vi "FFT and Power Spectrum Units.vi"() -> ()   [LabVIEW 2020]
doc: "This is an interactive example which allows you to explore the subject of FFT and spectrum output units.\n\nThe input signal to the FFT-based VIs is constructed as a single frequency component with a DC offset so that both the DC and non-DC amplitudes can be easily verified."
uses:
  <vilib>/measure/maspectr.llb/Power Spectrum and PSD Export Mode.ctl
  <vilib>/Analysis/2dsp.llb/Real FFT.vi
  <vilib>/Analysis/2dsp.llb/Power Spectrum (DBL).vi
  <vilib>/measure/maspectr.llb/FFT Power Spectrum and PSD for 1 Chan.vi
  <vilib>/measure/maspectr.llb/FFT Spectrum (Mag-Phase) for 1 Chan.vi
  <vilib>/measure/maspectr.llb/FFT Spectrum (Real-Im) for 1 Chan.vi
  <vilib>/Analysis/NI_AALPro.lvlib
  <vilib>/gmath/NI_Gmath.lvlib
  <vilib>/measure/NI_MAPro.lvlib
  <vilib>/measure/NI_MABase.lvlib
panel:
  in  "Instructions":string="Overview: Shows the propagation of units through FFT-based measurements. \nRequirements: LabVIEW Full Development System\nInstructions:\n1. Run the VI.  Make sure sine frequency is \"on bin\" by making sure it is an integer multiple of df = sample rate/number of samples.\n2. In the spectrum units table, click in either the Unit (DC) column or the Unit (freq > 0) column of any function row to validate agreement between the text formula in the cell and the spectral plot component.\n3. Click Stop to stop the VI."
  out "axis dx":dbl=1.0
  in  "x axis unit":u16(ring) items=["bin index", "frequency in Hz"]
  out "phase[k] in deg":dbl=-89.99999999994303
  out "phase spectrum":dbl[](array[numeric])
  out "k = bin index = f/df":dbl=10.0
  out "df (Hz) = Fs/N":dbl=20.0
  in  "Stop":bool
  in  "V":dbl=2.0
  out "spectrum units table":string[][](table)=[["FFT", "N * V", "N/2 * Vpk"], ["Power Spectrum", "V^2", "1/2 * Vrms^2"], ["Auto Power Spectrum", "V^2", "Vrms^2"], ["Amplitude and Phase Spectrum", "V", "Vrms"], ["FFT Power Spectrum", "V^2", "Vrms^2"], ["FFT Power Spectral Density", "V^2/Hz", "Vrms^2/Hz"], ["FFT Spectrum (Mag-Phase)", "V", "Vrms"], ["FFT Spectrum (Real-Imag)", "V", "Vrms"]]
  out "Vrms":dbl=2.1213203435596424
  out "X[0 or k]":dbl=150.0
  out "spectral plot":cluster{"t":dbl, "t":dbl, "magnitude":dbl[]}(graph)={"t"=0.0, "t"=1.0, "magnitude"=[]}
  out "time domain signal":waveform(dbl)(graph)={"t0"=timestamp(14.25 s since 1904-01-01), "dt"=0.0005, "Y"=[]}
  in  "Fs, sample rate":dbl=2000.0
  in  "N":dbl=100.0
  in  "sine frequency":dbl=200.0
  in  "Vpk":dbl=3.0
  # "Selecting either of the Unit columns in the table will place a cursor on the corresponding component in the plot, and the Y value of that component is displayed in the X[0 or k] indicator below."
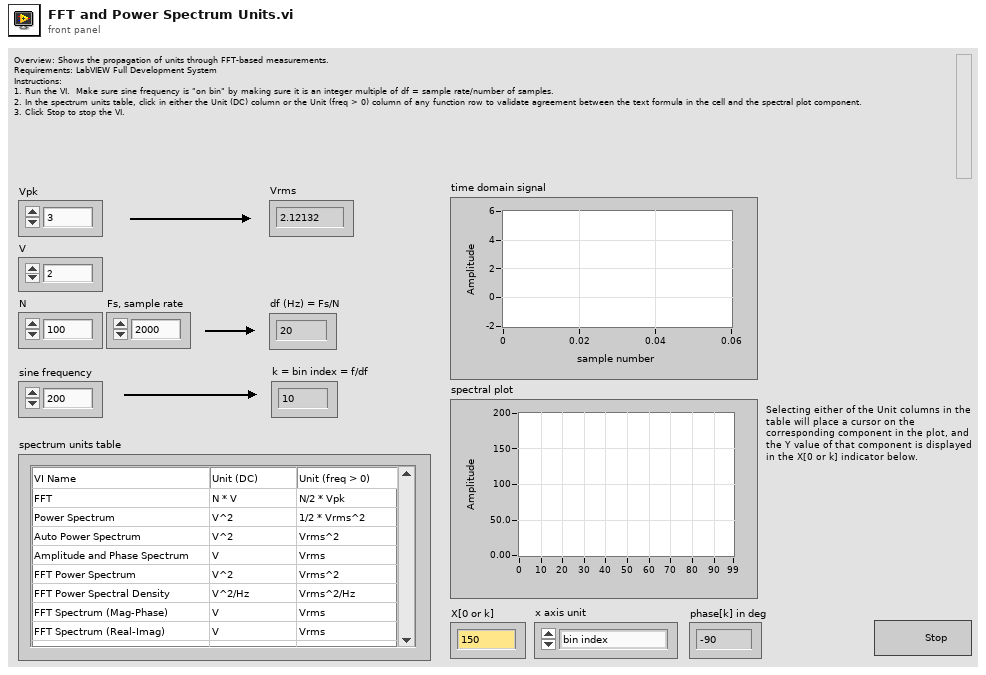
[diagram p1: front panel]
types:
  T1 = enum16{"None ", "Hanning", "Hamming", "Blackman-Harris", "Exact Blackman", "Blackman", "Flat Top", "4 Term B-Harris ", "7 Term B-Harris", "Low Sidelobe"}
  T2 = cluster{"dB On (F)":bool, "unwrap phase (F)":bool, "convert to degree (F)":bool}
  T3 = typedef "LVRowAndColumnTypeDef.ctl" = cluster{"Row":i32, "Column":i32}
  T4 = typedef "NI_MAPro.lvlib/Power Spectrum and PSD Export Mode.ctl" = u16
  T5 = cluster{"f0":dbl, "df":dbl, "imaginary part":dbl[]}
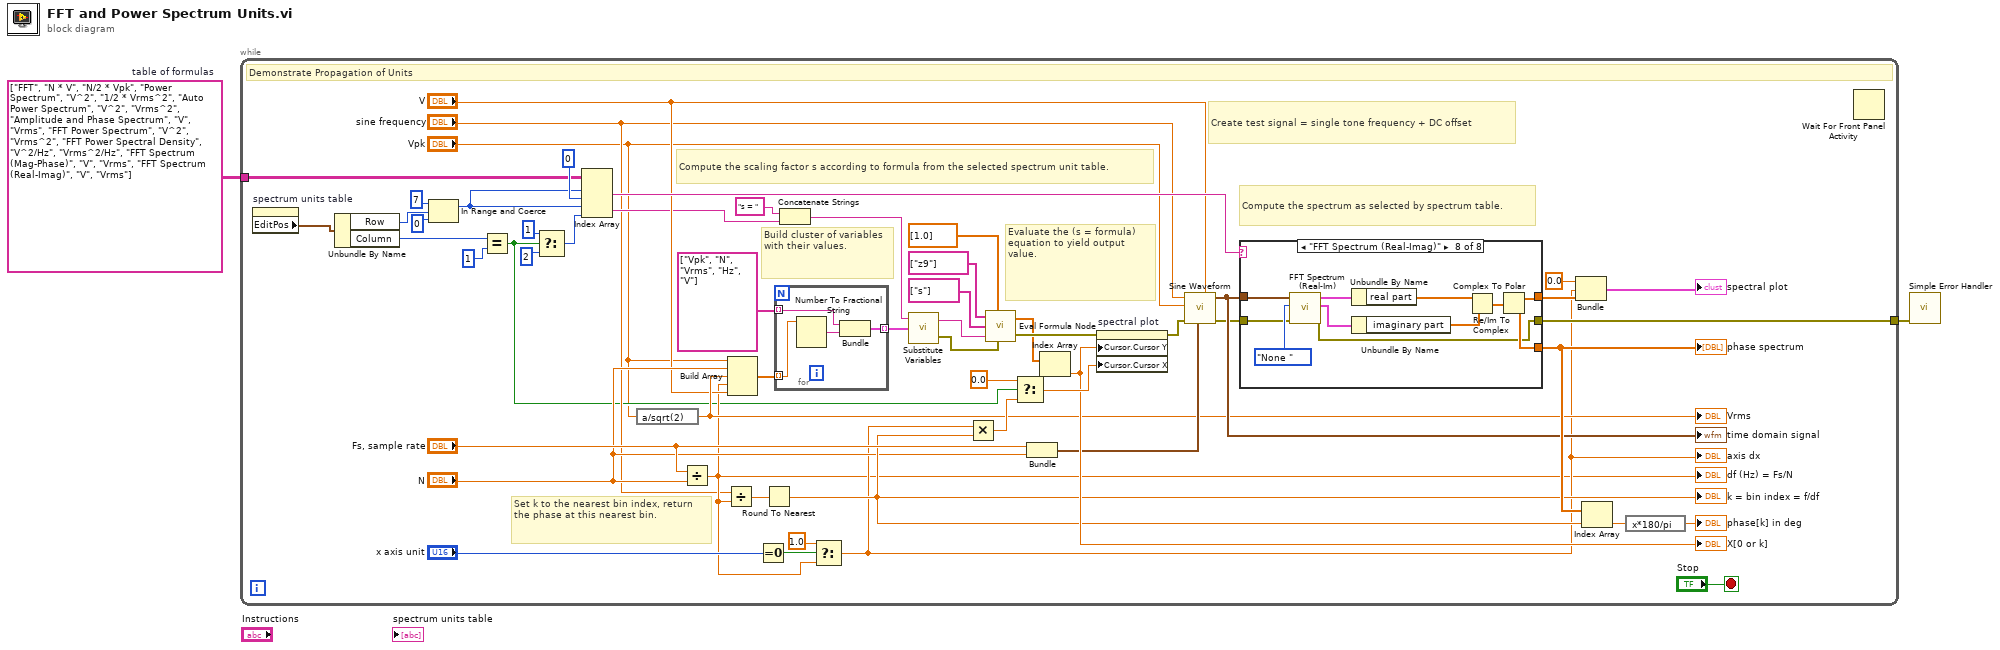
[diagram p0: block diagram]
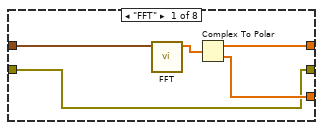
[diagram p2: hidden frame]
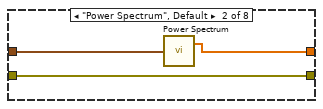
[diagram p3: hidden frame]
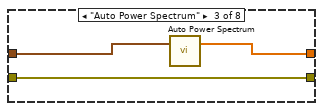
[diagram p4: hidden frame]
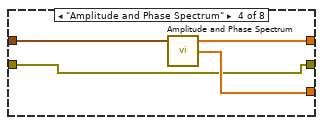
[diagram p5: hidden frame]
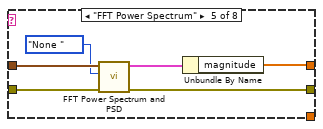
[diagram p6: hidden frame]
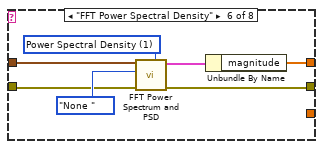
[diagram p7: hidden frame]
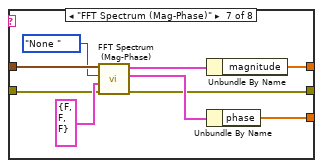
[diagram p8: hidden frame]
diagram:
  w1 = string[][] [["FFT", "N * V", "N/2 * Vpk"], ["Power Spectrum", "V^2", "1/2 * Vrms^2"], ["Auto Power Spectrum", "V^2", "Vrms^2"], ["Amplitude and Phase Spectrum", "V", "Vrms"], ["FFT Power Spectrum", "V^2", "Vrms^2"], ["FFT Power Spectral Density", "V^2/Hz", "Vrms^2/Hz"], ["FFT Spectrum (Mag-Phase)", "V", "Vrms"], ["FFT Spectrum (Real-Imag)", "V", "Vrms"]]  # table of formulas
  n1 = while {
    tunnel: [w13] -> w2
    tunnel: w1 -> [w3]
    stop <- "Stop" stop-if-true
    # "Build cluster of variables with their values."
    # "Set k to the nearest bin index, return the phase at this nearest bin."
    # "Compute the spectrum as selected by spectrum table."
    # "Create test signal = single tone frequency + DC offset"
    # "Evaluate the (s = formula) equation to yield output value."
    # "Compute the scaling factor s according to formula from the selected spectrum unit table."
    # "Demonstrate Propagation of Units"
    n2 = property on="spectrum units table" class="Tbl (strict)"() -> ("EditPos"=w57:T3)  [unwired: 2 in, 2 out]
    n3 = Unbundle By Name(w57) -> ("Row"=w54:i32, "Column"=w32:i32)
    n4 = In Range and Coerce(upper limit=7, x=w54, lower limit=0 ("y")) -> (coerced(x)=w14:i32)  [unwired: 1 out]
    n5 = Equal?(x=w32, y=1) -> (x = y?=w6:bool)
    n6 = Select(t=1, s=w6, f=2 ("t")) -> (s? t:f=w11:i32)
    n7 = Index Array(array=w3, index (row) #1=w14, index (col) #1=0 ("disabled index (col)"), index (row) #2=w14, index (col) #2=w11) -> (element #1=w28:string, element #2=w12:string)
    n8 = expression code="a/sqrt(2)"("Vpk") -> (w16:dbl)
    "Vrms" <- w16
    n9 = Divide(x="Fs, sample rate", y="N") -> (x/y=w8:dbl)
    "df (Hz) = Fs/N" <- w8
    n10 = Divide(x="sine frequency", y=w8) -> (x/y=w21:dbl)
    n11 = Build Array("Vpk", "N", w16, w8, "V") -> (w18:dbl[])
    n12 = Equal To 0?(x="x axis unit") -> (x = 0?=w26:bool)
    n13 = Round To Nearest(number=w21) -> (nearest integer value=w30:dbl)
    "k = bin index = f/df" <- w30
    n14 = for {
      tunnel: [w109] -> w36 mode=indexing
      tunnel: string[] ["Vpk", "N", "Vrms", "Hz", "V"] -> [w107] mode=indexing
      tunnel: w18 -> [w110] mode=indexing
      # "Build cluster of variables with their values"
      n15 = Number To Fractional String(number=w110) -> (F-format string=w108:string)  [unwired: 3 in]
      n16 = Bundle(w107, w108) -> (w109:cluster{string, string})  [unwired: 1 in]
    }
    n17 = Concatenate Strings("s = " ("string"), w12) -> (w44:string)
    n18 = Select(t=1.0, s=w26, f=w8) -> (s? t:f=w9:dbl)
    "axis dx" <- w9
    n19 = call <vilib>:"Substitute Variables.vi"("Substitution Rules"=w36, "original formula"=w44) -> ("error out"=w5:errorcluster, "formula after substitution"=w35:string)  [unwired: 1 in]
    n20 = Multiply(x=w9, y=w30) -> (x*y=w46:dbl)
    n21 = call <vilib>:"Eval Formula Node.vi"("Variables Input"=string[] ["z9"], "Input Values"=dbl[] [1.0], "Variables Output"=string[] ["s"], "formula"=w35, "error in (no error)"=w5) -> ("Output Values"=w40:dbl[], "error out"=w47:errorcluster)
    n22 = Select(t=0.0, s=w6, f=w46) -> (s? t:f=w42:dbl)
    n23 = Bundle("Fs, sample rate"="Fs, sample rate", "N"="N") -> (w27:cluster{"Fs, sample rate":dbl, "N":dbl})  [unwired: 1 in]
    n24 = Index Array(array=w40) -> (element=w31:dbl)  [unwired: 1 in]
    "X[0 or k]" <- w31
    n25 = property on="spectral plot" class="WFGraph (strict)"(error in=w47, "Cursor.Cursor Y"=w31, "Cursor.Cursor X"=w42) -> (error out=w10:errorcluster)  [unwired: 1 in, 1 out]
    n26 = call <vilib>:"Sine Waveform.vi"("offset"="V", "sampling info"=w27, "error in (no error)"=w10, "amplitude"="Vpk", "frequency"="sine frequency") -> ("error out"=w22:errorcluster, "signal out"=w49:waveform(dbl))  [unwired: 5 in]
    "time domain signal" <- w49
    n27 = case shown="\"FFT Spectrum (Real-Imag)\"" w28 {
      tunnel: [w61 w66 w68 w72 w77 w84 w93 w99] -> w23
      tunnel: w49 -> [w63 w65 w69 w73 w79 w86 w95 w106]
      tunnel: [w60 _ _ w71 _ _ w90 w98] -> w50
      tunnel: w22 -> [w59 w64 w67 w70 w75 w81 w88 w97]
      tunnel: [w59 w64 w67 w70 w74 w80 w87 w96] -> w13
      frame "FFT" {
        n28 = call-poly <vilib>:"FFT.vi"("X"=w63) -> ("FFT {X}"=w62:cdb[])  [unwired: 9 in, 1 out]
        n29 = Complex To Polar(r * e^(i*theta)=w62) -> (r=w61:dbl[], theta=w60:dbl[])
      }
      frame "Power Spectrum", Default {
        n30 = call-poly <vilib>:"Power Spectrum.vi"("X"=w65) -> ("Power Spectrum"=w66:dbl[])  [unwired: 1 out]
      }
      frame "Auto Power Spectrum" {
        n31 = call <vilib>:"Auto Power Spectrum.vi"("Signal (V)"=w69) -> ("Power Spectrum (V^2 rms)"=w68:dbl[])  [unwired: 1 in, 1 out]
      }
      frame "Amplitude and Phase Spectrum" {
        n32 = call <vilib>:"Amplitude and Phase Spectrum.vi"("Signal (V)"=w73) -> ("Amp Spectrum Phase (radians)"=w71:dbl[], "Amp Spectrum Mag (Vrms)"=w72:dbl[])  [unwired: 2 in, 1 out]
      }
      frame "FFT Power Spectrum" {
        n33 = call-poly <vilib>:"FFT Power Spectrum and PSD.vi"("error in (no error)"=w75, "window"=T1."None ", "time signal"=w79) -> ("error out"=w74:errorcluster, "Power Spectrum / PSD"=w78:cluster{"f0":dbl, "df":dbl, "magnitude":dbl[]})  [unwired: 5 in, 2 out]
        n34 = Unbundle By Name(w78) -> ("magnitude"=w77:dbl[])
      }
      frame "FFT Power Spectral Density" {
        w82 = T4 1 items=["Power Spectrum", "Power Spectral Density"] ("export mode")
        n35 = call-poly <vilib>:"FFT Power Spectrum and PSD.vi"("export mode"=w82, "error in (no error)"=w81, "window"=T1."None ", "time signal"=w86) -> ("error out"=w80:errorcluster, "Power Spectrum / PSD"=w85:cluster{"f0":dbl, "df":dbl, "magnitude":dbl[]})  [unwired: 4 in, 2 out]
        n36 = Unbundle By Name(w85) -> ("magnitude"=w84:dbl[])
      }
      frame "FFT Spectrum (Mag-Phase)" {
        n37 = call-poly <vilib>:"FFT Spectrum (Mag-Phase).vi"("error in (no error)"=w88, "view"=T2 {"dB On (F)"=FALSE, "unwrap phase (F)"=FALSE, "convert to degree (F)"=FALSE}, "window"=T1."None ", "time signal"=w95) -> ("error out"=w87:errorcluster, "phase"=w91:cluster{"f0":dbl, "df":dbl, "phase":dbl[]}, "magnitude"=w94:cluster{"f0":dbl, "df":dbl, "magnitude":dbl[]})  [unwired: 3 in, 2 out]
        n38 = Unbundle By Name(w94) -> ("magnitude"=w93:dbl[])
        n39 = Unbundle By Name(w91) -> ("phase"=w90:dbl[])
      }
      frame "FFT Spectrum (Real-Imag)" {
        n40 = call-poly <vilib>:"FFT Spectrum (Real-Im).vi"("error in (no error)"=w97, "window"=T1."None ", "time signal"=w106) -> ("error out"=w96:errorcluster, "imaginary part"=w103:T5, "real part"=w105:cluster{"f0":dbl, "df":dbl, "real part":dbl[]})  [unwired: 4 in, 2 out]
        n41 = Unbundle By Name(w105) -> ("real part"=w102:dbl[])
        n42 = Unbundle By Name(w103) -> ("imaginary part"=w101:dbl[])
        n43 = Re/Im To Complex(1:w101, 2:w102) -> (0:w100:cdb[])
        n44 = Complex To Polar(r * e^(i*theta)=w100) -> (r=w99:dbl[], theta=w98:dbl[])
      }
    }
    "phase spectrum" <- w50
    n45 = Bundle("t"=0.0, "t"=w9, "magnitude"=w23) -> (→"spectral plot":cluster{"t":dbl, "t":dbl, "magnitude":dbl[]})  [unwired: 1 in]
    n46 = Index Array(array=w50, index=w30) -> (element=w20:dbl)
    n47 = expression code="x*180/pi"(w20) -> (→"phase[k] in deg":dbl)
    n48 = Wait For Front Panel Activity() -> ()  [unwired: 3 in, 1 out]
  }
  n49 = call <vilib>:"Simple Error Handler.vi"("error in (no error)"=w2) -> ()  [unwired: 4 in, 5 out]
